vi "Read Proccess Error.vi"(8 "error in (no error)":errorcluster, 11 "Process State Data in":refnum<class "Process State Data.lvclass">) -> (0 "error out":errorcluster, 2 "Proccess Error":errorcluster, 3 "Process State Data out":refnum<class "Process State Data.lvclass">)   [LabVIEW 2022 SP3, in "Process State Data.lvclass"]
uses:
  Process State Data.lvclass
  Process State Data.lvclass/Process State Data.ctl
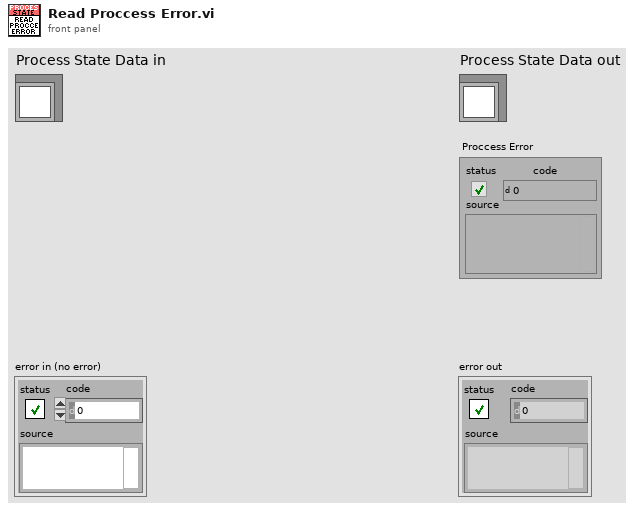
[diagram p1: front panel]
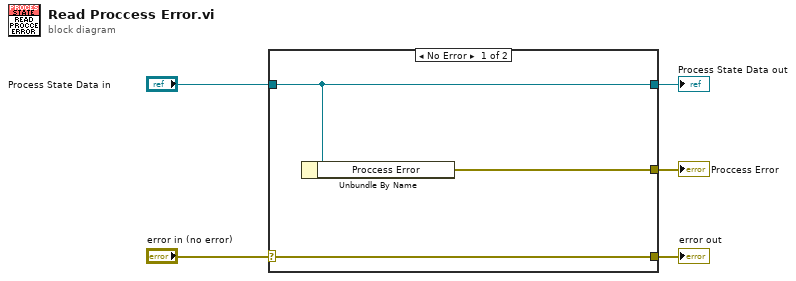
[diagram p0: block diagram]
diagram:
  n1 = case shown="No Error" "error in (no error)" {
    selector: "error in (no error)" -> [w8 w9]
    tunnel: [w8 w9] -> w4
    tunnel: [w7 w10] -> w2
    tunnel: "Process State Data in" -> [w7 w10]
    tunnel: [w6 _] -> w1
    frame No Error {
      n2 = Unbundle By Name(w7) -> ("Proccess Error"=w6:errorcluster)
    }
    frame Error {
    }
  }
  "error out" <- w4
  "Process State Data out" <- w2
  "Proccess Error" <- w1
